vi "Check Process2.vi"() -> ()   [LabVIEW 2018]
uses:
  F:/2222222222222222222/55W/ATE_Program20201119/API_Salcomp_CMES/CMESAPI.dll
  55W/ATE_Program20201119/API_Salcomp_CMES/CMESAPI.dll
panel:
  out "CheckRouteForSerialNumber":bool
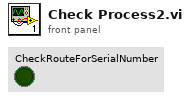
[diagram p1: front panel]
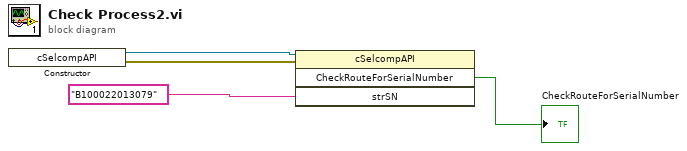
[diagram p0: block diagram]
diagram:
  n1 = constructor class="cSelcompAPI"() -> (reference out=w4:refnum<k24>, error out=w1:errorcluster)  [unwired: 3 in, 1 out]
  n2 = invoke class="cSelcompAPI" method="CheckRouteForSerialNumber"(reference=w4, error in=w1, "strSN"="B100022013079" ("serialNumber")) -> ("CheckRouteForSerialNumber"=→"CheckRouteForSerialNumber":bool)  [unwired: 1 in, 3 out]
